vi "Write Operator.vi"(8 "error in (no error)":errorcluster, 10 "External Calibration Operator":refnum<class "External Calibration Operator.lvclass">, 11 "Asset External Calibration in":refnum<class "Asset External Calibration.lvclass">) -> (0 "error out":errorcluster, 3 "Asset External Calibration out":refnum<class "Asset External Calibration.lvclass">)   [LabVIEW 2019, in "Asset External Calibration.lvclass"]
uses:
  Asset External Calibration.lvclass
  External Calibration Operator/External Calibration Operator.lvclass
  Asset External Calibration.lvclass/Asset External Calibration.ctl
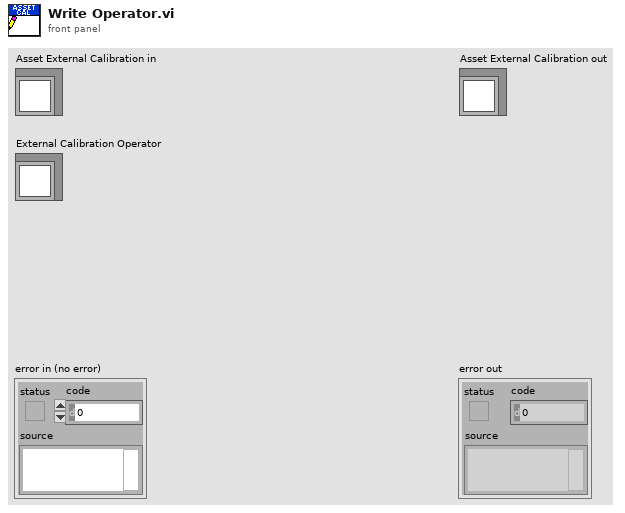
[diagram p1: front panel]
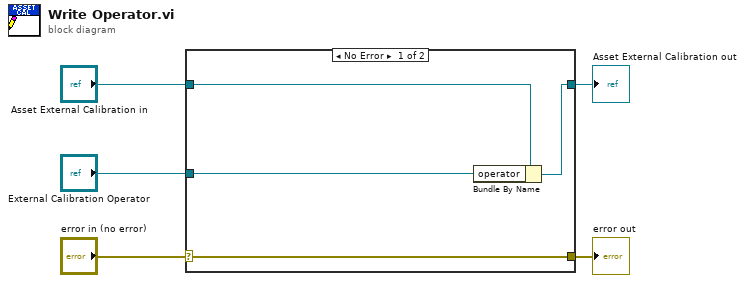
[diagram p0: block diagram]
diagram:
  n1 = case shown="No Error" "error in (no error)" {
    selector: "error in (no error)" -> [w9 w10]
    tunnel: [w9 w10] -> w4
    tunnel: [w7 w11] -> w2
    tunnel: "Asset External Calibration in" -> [w8 w11]
    tunnel: "External Calibration Operator" -> [w6 _]
    frame No Error {
      n2 = Bundle By Name(cluster=w8, "operator"=w6) -> (w7:refnum<class "Asset External Calibration.lvclass">)
    }
    frame Error {
    }
  }
  "error out" <- w4
  "Asset External Calibration out" <- w2
